vi "Harvard Apparatus PHD Ultra Series Push Button.vi"() -> ()   [LabVIEW 2018]
doc: "Demonstrates interactive control on the pump. User can interactively control the operation on the pump such as infuse, pause, withdraw and stop. \nThis VI continously output the status and the delivered volume.\n\n<b>Note:</b>\n- The pump does not support remote syringe volume setting. User must set the syringe volume on the pump before running this example. The Target Volume must be less than or equal to the syringe volume. \n- Does not work with Serial Interface. Delays need to be added for Serial Interface."
uses:
  <instrlib>/Harvard Apparatus PHD Ultra Series/Harvard Apparatus PHD Ultra Series.lvlib
panel:
  out "Infused Volume":dbl
  out "Withdrawn Volume":dbl
  out "Infuse Units":u16(ring)=1 items=["milliliters", "microliters", "nanoliters", "picoliters"]
  out "Withdraw Units":u16(ring)=1 items=["milliliters", "microliters", "nanoliters", "picoliters"]
  in  "# Syringes":i32=1
  in  "stop":bool
  in  "Syringe Diameter (20 mm)":dbl=44.0 min=1.0 max=99.0 format="%#.3f"
  in  "Tab Control":enum32{"Steady", "Ramp"}(tab)
  in  "Flow Rate (5)":dbl=5.0 format="%#.4f"
  in  "Flow Rate Units (1:ml/min)":u32(ring)=1 items=["milliliters per hour (ml/hr)", "milliliters per minute (ml/min)", "milliliters per second (ml/sec)", "microliters per hour (ul/hr)", "microliters per minute (ul/min)", "microliters per second (ul/sec)", "nanoliters per hour (nl/hr)", "nanoliters per minute (nl/min)", "nanoliters per second (nl/sec)", "picoliters per hour (pl/hr)", "picoliters per minute (pl/min)", "picoliters per second (pl/sec)"]
  in  "Pause":bool
  in  "Start":bool
  in  "Run Method (0:Infuse)":u16(ring)=1 items=["Infuse", "Withdraw"]
  in  "Initial Flow Rate (5.00)":dbl=5.0 format="%#.4f"
  in  "Pump Direction (0:Infuse)":u16(ring)=1 items=["Infuse", "Withdraw"]
  in  "Infuse Time":dbl=5.0 format="%#.4f"
  in  "Final Flow Rate (5.00)":dbl=50.0 format="%#.4f"
  in  "Flow Rate Units (1:ml/min) 2":u32(ring)=1 items=["milliliters per hour (ml/hr)", "milliliters per minute (ml/min)", "milliliters per second (ml/sec)", "microliters per hour (ul/hr)", "microliters per minute (ul/min)", "microliters per second (ul/sec)", "nanoliters per hour (nl/hr)", "nanoliters per minute (nl/min)", "nanoliters per second (nl/sec)", "picoliters per hour (pl/hr)", "picoliters per minute (pl/min)", "picoliters per second (pl/sec)"]
  in  "Start Ramp":bool
  in  "Baud Rate (115200)":u32(ring)=115200 items=["9600"=9600, "19200"=19200, "38400"=38400, "57600"=57600, "115200"=115200]
  out "Idle":bool
  out "Withdrawing":bool
  out "Infusing":bool
  in  "Stop":bool
  in  "VISA resource name":refnum<visa-resource-name>="COM25"
  # "NOTE: The flow rate is compensated for the number of syringes in the code"
  # "Status"
  # "Controls"
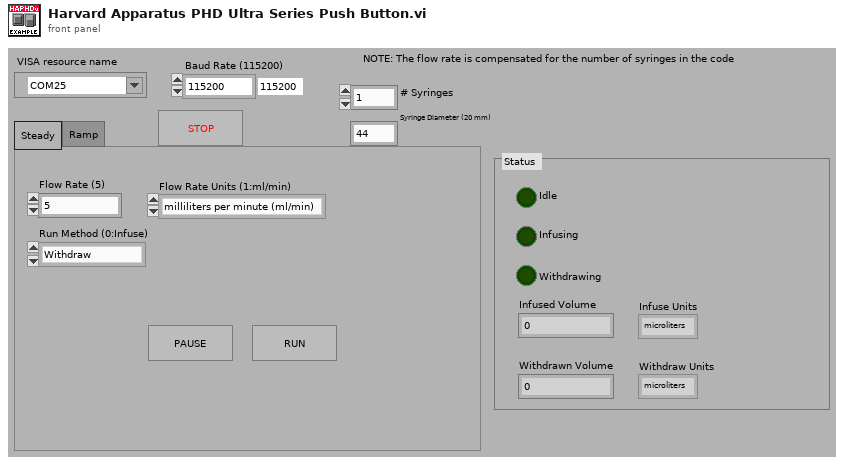
[diagram p1: front panel]
types:
  T1 = enum16{"open", "open or create", "create or replace", "create", "open (read-only)"}
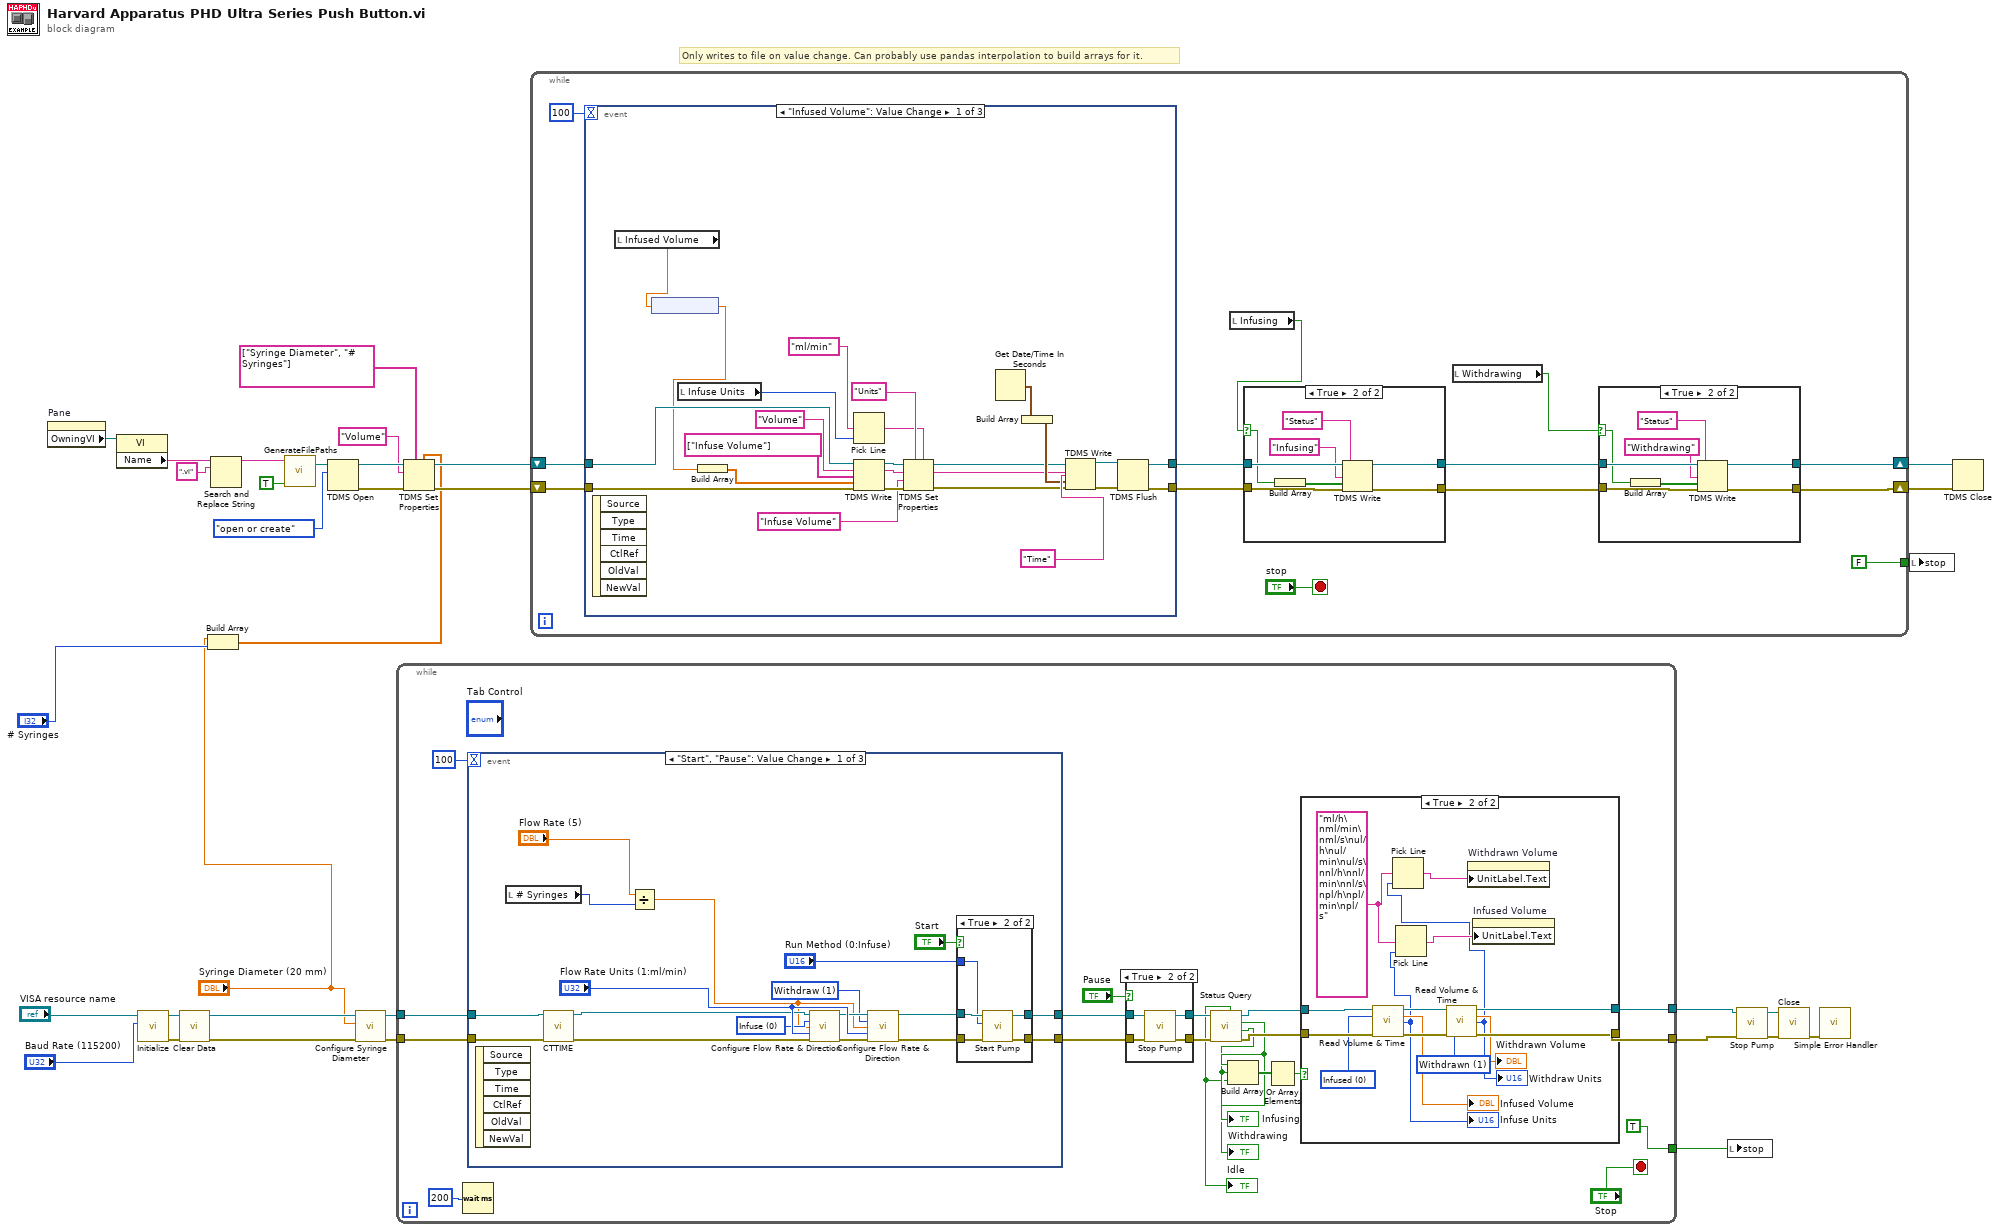
[diagram p0: block diagram]
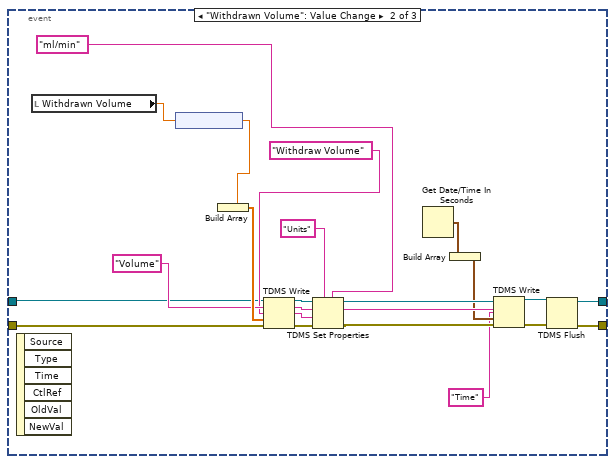
[diagram p4: hidden frame]
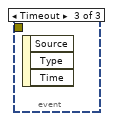
[diagram p5: hidden frame]
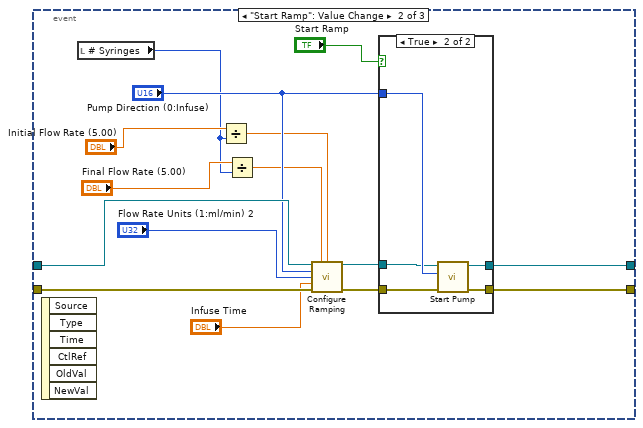
[diagram p9: hidden frame]
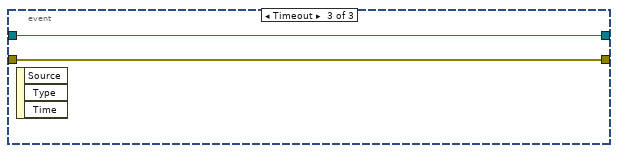
[diagram p11: hidden frame]
diagram:
  # "Only writes to file on value change. Can probably use pandas interpolation to build arrays for it."
  n1 = property on="Pane" class="Pane"() -> ("OwningVI"=w20:refnum<vi>)  [unwired: 2 in, 2 out]
  n2 = property class="VI"(reference=w20) -> ("Name"=w16:string)  [unwired: 1 in, 2 out]
  n3 = call <instrlib>:"Initialize.vi"("Baud Rate (115200)"="Baud Rate (115200)", "VISA resource name"="VISA resource name") -> ("error out"=w32:errorcluster, "VISA resource name out"=w31:refnum<visa-resource-name>)  [unwired: 8 in]
  n4 = call <instrlib>:"Clear Data.vi"("error in (no error)"=w32, "VISA resource name"=w31) -> ("error out"=w29:errorcluster, "VISA resource name out"=w30:refnum<visa-resource-name>)  [unwired: 8 in]
  n5 = Build Array("Syringe Diameter (20 mm)", "# Syringes") -> (w1:dbl[])
  n6 = Search and Replace String(input string=w16, search string=".vi") -> (result string=w18:string)  [unwired: 6 in, 3 out]
  n7 = call "GenerateFilePaths.vi"("Logfile? (F)"=TRUE ("Logfile?"), "Device Name"=w18) -> ("Path"=w15:path)  [unwired: 3 in]
  n8 = TDMS Open(10:T1."open or create" ("operation (0:open)"), 11:w15) -> (0:w9:errorcluster, 3:w8:refnum<k34>)  [unwired: 5 in]
  n9 = call <instrlib>:"Configure Syringe Diameter.vi"("error in (no error)"=w29, "Syringe Diameter (20 mm)"="Syringe Diameter (20 mm)", "VISA resource name"=w30) -> ("error out"=w21:errorcluster, "VISA resource name out"=w22:refnum<visa-resource-name>)  [unwired: 7 in]
  n10 = while {
    tunnel: w22 -> [w53]
    tunnel: [w42] -> w25
    tunnel: [w41] -> w24
    tunnel: w21 -> [w50]
    tunnel: [TRUE] -> w11
    stop <- "Stop" stop-if-true
    n11 = Wait (ms)(milliseconds to wait=u32 200) -> ()  [unwired: 1 out]
    n12 = event shown="[0] \"Start\", \"Pause\": Value Change" {
      selector: _ -> [_ _ _]
      dyn-events: _ -> [_ _ _]
      timeout: 100 -> [_ _ _]
      tunnel: w50 -> [w81 w112 w124]
      tunnel: w53 -> [w83 w113 w125]
      tunnel: [w93 w115 w125] -> w49
      tunnel: [w92 w114 w124] -> w48
      event "Start", "Pause": Value Change {
        w86 = u16 0 items=["Infuse", "Withdraw"] ("Pump Method (0:Infuse)")
        w87 = u16 1 items=["Infuse", "Withdraw"] ("Pump Method (0:Infuse)")
        n13 = event-data() -> ()  [unwired: 1 in, 6 out]
        n14 = local read "# Syringes"() -> (w78:i32)
        n15 = call <instrlib>:"CTTIME.vi"("VISA resource name"=w83, "error in (no error)"=w81) -> ("VISA resource name out"=w82:refnum<visa-resource-name>, "error out"=w80:errorcluster)  [unwired: 12 in]
        n16 = Divide(x="Flow Rate (5)", y=w78) -> (x/y=w77:dbl)
        n17 = call <instrlib>:"Configure Flow Rate & Direction.vi"("VISA resource name"=w82, "Pump Direction (0:Infuse)"=w86, "Flow Rate (5.00)"=w77, "Flow Rate Units (1:ml/min)"="Flow Rate Units (1:ml/min)", "error in (no error)"=w80) -> ("VISA resource name out"=w88:refnum<visa-resource-name>, "error out"=w90:errorcluster)  [unwired: 9 in]
        n18 = call <instrlib>:"Configure Flow Rate & Direction.vi"("VISA resource name"=w88, "Pump Direction (0:Infuse)"=w87, "Flow Rate (5.00)"=w77, "Flow Rate Units (1:ml/min)"="Flow Rate Units (1:ml/min)", "error in (no error)"=w90) -> ("VISA resource name out"=w85:refnum<visa-resource-name>, "error out"=w84:errorcluster)  [unwired: 9 in]
        n19 = case shown="True" "Start" {
          tunnel: w85 -> [w96 w101]
          tunnel: w84 -> [w95 w100]
          tunnel: [w96 w99] -> w93
          tunnel: [w95 w98] -> w92
          tunnel: "Run Method (0:Infuse)" -> [_ w97]
          frame False {
          }
          frame True {
            n20 = call <instrlib>:"Start Pump.vi"("error in (no error)"=w100, "Run Direction (0:Infuse)"=w97, "VISA resource name"=w101) -> ("error out"=w98:errorcluster, "VISA resource name out"=w99:refnum<visa-resource-name>)  [unwired: 7 in]
          }
        }
      }
      event "Start Ramp": Value Change {
        n21 = event-data() -> ()  [unwired: 1 in, 6 out]
        n22 = local read "# Syringes"() -> (w102:i32)
        n23 = Divide(x="Initial Flow Rate (5.00)", y=w102) -> (x/y=w103:dbl)
        n24 = Divide(x="Final Flow Rate (5.00)", y=w102) -> (x/y=w104:dbl)
        n25 = call <instrlib>:"Configure Ramping.vi"("VISA resource name"=w113, "End Rate (10.00)"=w104, "Start Rate (5.00)"=w103, "Pump Method (0:Infuse)"="Pump Direction (0:Infuse)", "Flow Rate Units (1:ml/min)"="Flow Rate Units (1:ml/min) 2", "Ramp Time (10 seconds)"="Infuse Time", "error in (no error)"=w112) -> ("VISA resource name out"=w110:refnum<visa-resource-name>, "error out"=w111:errorcluster)  [unwired: 7 in]
        n26 = case shown="True" "Start Ramp" {
          tunnel: "Pump Direction (0:Infuse)" -> [_ w123]
          tunnel: w110 -> [w118 w122]
          tunnel: w111 -> [w117 w121]
          tunnel: [w118 w120] -> w115
          tunnel: [w117 w119] -> w114
          frame False {
          }
          frame True {
            n27 = call <instrlib>:"Start Pump.vi"("error in (no error)"=w121, "Run Direction (0:Infuse)"=w123, "VISA resource name"=w122) -> ("error out"=w119:errorcluster, "VISA resource name out"=w120:refnum<visa-resource-name>)  [unwired: 7 in]
          }
        }
      }
      event Timeout {
        n28 = event-data() -> ()  [unwired: 1 in, 3 out]
      }
    }
    n29 = case shown="True" "Pause" {
      tunnel: w49 -> [w72 w76]
      tunnel: w48 -> [w71 w75]
      tunnel: [w72 w74] -> w46
      tunnel: [w71 w73] -> w47
      frame False {
      }
      frame True {
        n30 = call <instrlib>:"Stop Pump.vi"("error in (no error)"=w75, "VISA resource name"=w76) -> ("error out"=w73:errorcluster, "VISA resource name out"=w74:refnum<visa-resource-name>)  [unwired: 8 in]
      }
    }
    n31 = call <instrlib>:"Status Query.vi"("error in (no error)"=w47, "VISA resource name"=w46) -> ("error out"=w40:errorcluster, "Withdrawing"=w35:bool, "Infusing"=w36:bool, "VISA resource name out"=w39:refnum<visa-resource-name>, "Idle"=w34:bool)  [unwired: 4 in, 1 out]
    "Infusing" <- w36
    "Withdrawing" <- w35
    "Idle" <- w34
    n32 = Build Array(w36, w35, w34) -> (w37:bool[])
    n33 = Or Array Elements(Boolean array=w37) -> (logical OR=w38:bool)
    n34 = case shown="True" w38 {
      tunnel: w40 -> [w54 w70]
      tunnel: w39 -> [w55 w69]
      tunnel: [w55 w68] -> w42
      tunnel: [w54 w67] -> w41
      frame False {
        # "Reads Volume only when the pump is infusing or withdrawing. This will reduce the commands sent to the instrument and prevents the instrument having errors."
      }
      frame True {
        w58 = "ml/h\nml/min\nml/s\nul/h\nul/min\nul/s\nnl/h\nnl/min\nnl/s\npl/h\npl/min\npl/s" ("multi-line string")
        w63 = u16 0 items=["Infused", "Withdrawn"] ("Pump Method (0:Infused)")
        w64 = u16 1 items=["Infused", "Withdrawn"] ("Pump Method (0:Infused)")
        n35 = call <instrlib>:"Read Volume & Time .vi"("VISA resource name"=w69, "Pump Direction (0:Infused)"=w63, "error in (no error)"=w70) -> ("VISA resource name out"=w65:refnum<visa-resource-name>, "Volume"=→"Infused Volume":dbl, "Volume Units"=w57:u16, "error out"=w66:errorcluster)  [unwired: 7 in, 2 out]
        "Infuse Units" <- w57
        n36 = Pick Line(multi-line string=w58, line index=w57) -> (output string=w59:string)  [unwired: 1 in]
        n37 = call <instrlib>:"Read Volume & Time .vi"("VISA resource name"=w65, "Pump Direction (0:Infused)"=w64, "error in (no error)"=w66) -> ("VISA resource name out"=w68:refnum<visa-resource-name>, "Volume"=→"Withdrawn Volume":dbl, "Volume Units"=w56:u16, "error out"=w67:errorcluster)  [unwired: 7 in, 2 out]
        "Withdraw Units" <- w56
        n38 = Pick Line(multi-line string=w58, line index=w56) -> (output string=w60:string)  [unwired: 1 in]
        n39 = property on="Withdrawn Volume" class="DigNum (strict)"("UnitLabel.Text"=w60) -> ()  [unwired: 2 in, 2 out]
        n40 = property on="Infused Volume" class="DigNum (strict)"("UnitLabel.Text"=w59) -> ()  [unwired: 2 in, 2 out]
      }
    }
  }
  n41 = TDMS Set Properties(5:w1, 7:string[] ["Syringe Diameter", "# Syringes"] ("group name in (Untitled)"), 8:w9, 10:"Volume" ("group name in (Untitled)"), 11:w8) -> (0:w6:errorcluster, 3:w7:refnum<k34>)  [unwired: 1 in, 2 out]
  n42 = while {
    shift-right: [w128] -> w13
    shift-left: w7 -> [w138]
    shift-right: [w129] -> w12
    shift-left: w6 -> [w137]
    tunnel: [FALSE] -> w10
    stop <- "stop" stop-if-true
    n43 = event shown="[0] \"Infused Volume\": Value Change" {
      selector: _ -> [_ _ _]
      dyn-events: _ -> [_ _ _]
      timeout: 100 -> [_ _ _]
      tunnel: w138 -> [w183 w190 _]
      tunnel: w137 -> [w182 w189 _]
      tunnel: [w180 w188 _] -> w133
      tunnel: [w179 w187 _] -> w132
      event "Infused Volume": Value Change {
        n44 = event-data() -> ()  [unwired: 1 in, 6 out]
        n45 = local read "Infused Volume"() -> (w160:dbl)
        n46 = node(w160) -> (w159:dbl[unit])
        n47 = local read "Infuse Units"() -> (w174:u16)
        n48 = Build Array(w159) -> (w162:dbl[unit][])
        n49 = Pick Line(multi-line string="ml/min", line index=w174) -> (output string=w175:string)  [unwired: 1 in]
        n50 = TDMS Write(0:w183, 5:"Volume" ("group name in (Untitled)"), 7:string[] ["Infuse Volume"], 9:w162, 11:w182) -> (4:w177:refnum<k34>, 6:w178:string, 15:w172:errorcluster)  [unwired: 1 in, 1 out]
        n51 = TDMS Set Properties(5:w175, 7:"Units", 8:w172, 9:"Infuse Volume" ("String"), 10:w178, 11:w177) -> (0:w164:errorcluster, 2:w163:string, 3:w165:refnum<k34>)  [unwired: 1 out]
        n52 = Get Date/Time In Seconds() -> (seconds since 1Jan1904=w167:timestamp)
        n53 = Build Array(w167) -> (w166:timestamp[])
        n54 = TDMS Write(0:w165, 5:w163, 7:"Time", 9:w166, 11:w164) -> (4:w170:refnum<k34>, 15:w169:errorcluster)  [unwired: 1 in, 2 out]
        n55 = TDMS Flush(4:w169, 7:w170) -> (0:w179:errorcluster, 3:w180:refnum<k34>)
      }
      event "Withdrawn Volume": Value Change {
        n56 = event-data() -> ()  [unwired: 1 in, 6 out]
        n57 = local read "Withdrawn Volume"() -> (w184:dbl)
        n58 = node(w184) -> (w185:dbl[unit])
        n59 = Build Array(w185) -> (w199:dbl[unit][])
        n60 = TDMS Write(0:w190, 5:"Volume" ("group name in (Untitled)"), 7:"Withdraw Volume", 9:w199, 11:w189) -> (4:w195:refnum<k34>, 6:w196:string, 8:w197:string, 15:w198:errorcluster)  [unwired: 1 in]
        n61 = TDMS Set Properties(5:"ml/min" ("multi-line string"), 7:"Units", 8:w198, 9:w197, 10:w196, 11:w195) -> (0:w206:errorcluster, 2:w205:string, 3:w204:refnum<k34>)  [unwired: 1 out]
        n62 = Get Date/Time In Seconds() -> (seconds since 1Jan1904=w202:timestamp)
        n63 = Build Array(w202) -> (w203:timestamp[])
        n64 = TDMS Write(0:w204, 5:w205, 7:"Time", 9:w203, 11:w206) -> (4:w200:refnum<k34>, 15:w201:errorcluster)  [unwired: 1 in, 2 out]
        n65 = TDMS Flush(4:w201, 7:w200) -> (0:w187:errorcluster, 3:w188:refnum<k34>)
      }
      event Timeout {
        n66 = event-data() -> ()  [unwired: 1 in, 3 out]
      }
    }
    n67 = local read "Infusing"() -> (w131:bool)
    n68 = case shown="True" w131 {
      selector: w131 -> [_ w153]
      tunnel: w133 -> [w150 w158]
      tunnel: w132 -> [w149 w157]
      tunnel: [w149 w156] -> w130
      tunnel: [w150 w155] -> w127
      frame False {
      }
      frame True {
        n69 = Build Array(w153) -> (w151:bool[])
        n70 = TDMS Write(0:w158, 5:"Status" ("group name in (Untitled)"), 7:"Infusing", 9:w151, 11:w157) -> (4:w155:refnum<k34>, 15:w156:errorcluster)  [unwired: 1 in, 2 out]
      }
    }
    n71 = local read "Withdrawing"() -> (w126:bool)
    n72 = case shown="True" w126 {
      selector: w126 -> [_ w143]
      tunnel: w127 -> [w140 w148]
      tunnel: w130 -> [w139 w147]
      tunnel: [w139 w146] -> w129
      tunnel: [w140 w145] -> w128
      frame False {
      }
      frame True {
        n73 = Build Array(w143) -> (w141:bool[])
        n74 = TDMS Write(0:w148, 5:"Status" ("group name in (Untitled)"), 7:"Withdrawing", 9:w141, 11:w147) -> (4:w145:refnum<k34>, 15:w146:errorcluster)  [unwired: 1 in, 2 out]
      }
    }
  }
  n75 = local write "stop"(w11) -> ()
  n76 = call <instrlib>:"Stop Pump.vi"("error in (no error)"=w24, "VISA resource name"=w25) -> ("error out"=w28:errorcluster, "VISA resource name out"=w27:refnum<visa-resource-name>)  [unwired: 8 in]
  n77 = call <instrlib>:"Close.vi"("error in (no error)"=w28, "VISA resource name"=w27) -> ("error out"=w26:errorcluster)  [unwired: 9 in]
  n78 = call <vilib>:"Simple Error Handler.vi"("error in (no error)"=w26) -> ()  [unwired: 4 in, 5 out]
  n79 = local write "stop"(w10) -> ()
  n80 = TDMS Close(8:w12, 11:w13) -> ()  [unwired: 2 out]
